vi "Add Default Enum.vi"(6 "Hdr Name":T1, 8 "error in (no error)":errorcluster, 9 "Enum Values":u16[](array[numeric]), 11 "Thermocouple in":refnum<class "Thermocouple.lvclass">) -> (0 "error out":errorcluster, 3 "Thermocouple out":refnum<class "Thermocouple.lvclass">)   [LabVIEW 2012, in "Measurement Channels.lvlib" / "Thermocouple.lvclass"]
uses:
  Thermocouple.lvclass
  Common/Controls/HeaderNames.ctl
  SubVIs Table/Custom Ctls Table/ge_ColType.ctl
  Thermocouple.lvclass/Thermocouple.ctl
  Class Channel/Write Unit_EU.vi
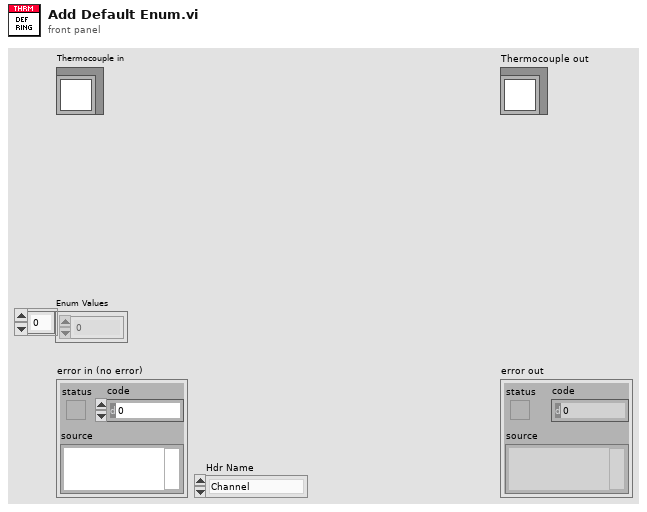
[diagram p1: front panel]
types:
  T1 = typedef "HeaderNames.ctl" = enum16{"Channel", "Device", "Spacer", "Description", "MB", "Range", "Terminal", "Coupling", "Thresh (V)", "Pulse/Rev", "Slope", "Min EU", "Min RPM", "mV/EU", "Iex", "Temp Units", "Type", "CJC Src", "CJC Val", "Ro", "Wire Cfg", "Strain Mode", "Vex", "Bridge Type", "GF", "Gauge Res", "Poisson", "Lead Res", "Init Strain", "GAF", "Scale", "Offset", "Unit (EU)", "dB?", "dB Ref", "Cal Mag", "Cal Units", "Max Temp", "Min Temp", "Max Strain", "Min Strain"}
  T2 = typedef "ge_ColType.ctl" = enum16{"Volts", "Amps", "Ohms", "TermCfg", "WireCfg", "Coup", "Slope", "Iex", "CalUnits", "ThrmUnits", "ThrmType", "CJCSrc", "BrdgType", "Strn Mode", "RTDType"}
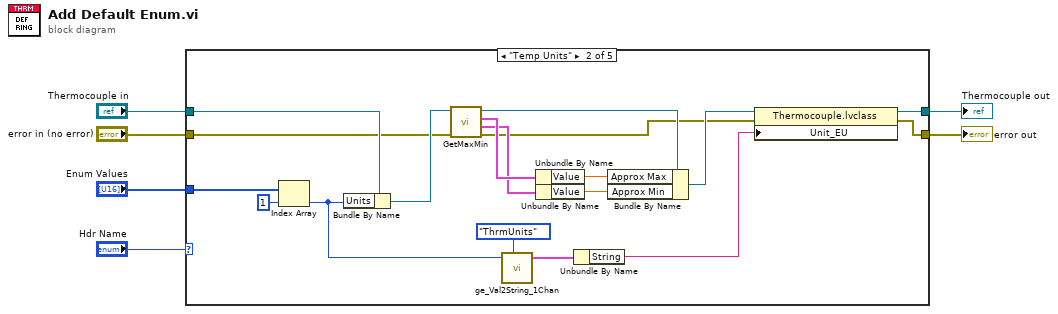
[diagram p0: block diagram]
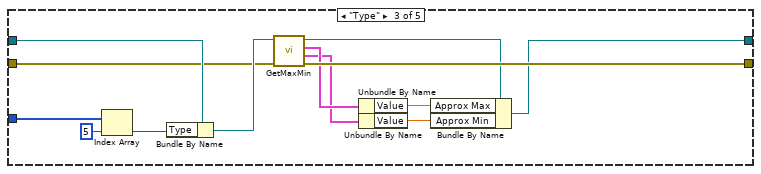
[diagram p3: hidden frame]
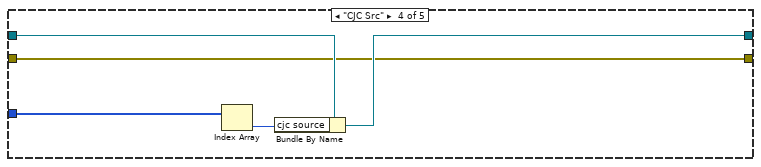
[diagram p4: hidden frame]
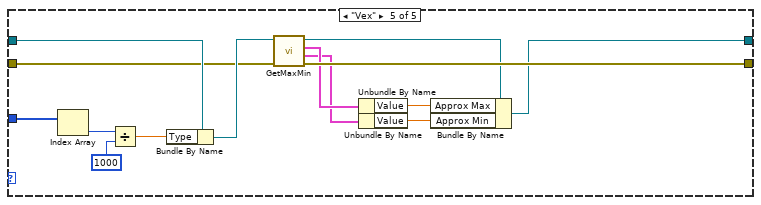
[diagram p5: hidden frame]
diagram:
  n1 = case shown="\"Temp Units\"" "Hdr Name" {
    tunnel: "Thermocouple in" -> [w8 w26 w39 w44 w58]
    tunnel: "error in (no error)" -> [w7 w24 w37 w40 w56]
    tunnel: [w8 w15 w33 w41 w53] -> w3
    tunnel: [w7 w14 w36 w40 w55] -> w2
    tunnel: "Enum Values" -> [_ w18 w28 w42 w46]
    frame Default {
    }
    frame "Temp Units" {
      n2 = Index Array(array=w18, index=1) -> (element=w10:u16)
      n3 = Bundle By Name(cluster=w26, "Units"=w10) -> (w25:refnum<class "Thermocouple.lvclass">)
      n4 = call-dynamic "GetMaxMin.vi"("error in (no error)"=w24, "Thermocouple in"=w25) -> ("error out"=w13:errorcluster, "Min"=w19:cluster{"Value":dbl, "Text":string}, "Max"=w22:cluster{"Value":dbl, "Text":string}, "Thermocouple out"=w23:refnum<class "Thermocouple.lvclass">)  [unwired: 6 in]
      n5 = call "ge_Val2String_1Chan.vi"("Value"=w10, "ColType"=ge_ColType."ThrmUnits") -> ("String and Val"=w11:cluster{"String":string, "Value":u16})  [unwired: 5 in]
      n6 = Unbundle By Name(w22) -> ("Value"=w21:dbl)
      n7 = Unbundle By Name(w19) -> ("Value"=w20:dbl)
      n8 = Unbundle By Name(w11) -> ("String"=w9:string)
      n9 = Bundle By Name(cluster=w23, "Approx Max"=w21, "Approx Min"=w20) -> (w16:refnum<class "Thermocouple.lvclass">)
      n10 = property class="Thermocouple.lvclass"(reference=w16, error in=w13, "Unit_EU"=w9) -> (reference out=w15:refnum<class "Thermocouple.lvclass">, error out=w14:errorcluster)
    }
    frame "Type" {
      n11 = Index Array(array=w28, index=5) -> (element=w35:u16)
      n12 = Bundle By Name(cluster=w39, "Type"=w35) -> (w38:refnum<class "Thermocouple.lvclass">)
      n13 = call-dynamic "GetMaxMin.vi"("error in (no error)"=w37, "Thermocouple in"=w38) -> ("error out"=w36:errorcluster, "Min"=w29:cluster{"Value":dbl, "Text":string}, "Max"=w32:cluster{"Value":dbl, "Text":string}, "Thermocouple out"=w34:refnum<class "Thermocouple.lvclass">)  [unwired: 6 in]
      n14 = Unbundle By Name(w32) -> ("Value"=w31:dbl)
      n15 = Unbundle By Name(w29) -> ("Value"=w30:dbl)
      n16 = Bundle By Name(cluster=w34, "Approx Max"=w31, "Approx Min"=w30) -> (w33:refnum<class "Thermocouple.lvclass">)
    }
    frame "CJC Src" {
      n17 = Index Array(array=w42) -> (element=w43:u16)  [unwired: 1 in]
      n18 = Bundle By Name(cluster=w44, "cjc source"=w43) -> (w41:refnum<class "Thermocouple.lvclass">)
    }
    frame "Vex" {
      n19 = Index Array(array=w46) -> (element=w48:u16)  [unwired: 1 in]
      n20 = Divide(x=w48, y=1000) -> (x/y=w45:dbl)
      n21 = Bundle By Name(cluster=w58, "Type"=w45) -> (w57:refnum<class "Thermocouple.lvclass">)
      n22 = call-dynamic "GetMaxMin.vi"("error in (no error)"=w56, "Thermocouple in"=w57) -> ("error out"=w55:errorcluster, "Min"=w49:cluster{"Value":dbl, "Text":string}, "Max"=w52:cluster{"Value":dbl, "Text":string}, "Thermocouple out"=w54:refnum<class "Thermocouple.lvclass">)  [unwired: 6 in]
      n23 = Unbundle By Name(w52) -> ("Value"=w51:dbl)
      n24 = Unbundle By Name(w49) -> ("Value"=w50:dbl)
      n25 = Bundle By Name(cluster=w54, "Approx Max"=w51, "Approx Min"=w50) -> (w53:refnum<class "Thermocouple.lvclass">)
    }
  }
  "error out" <- w2
  "Thermocouple out" <- w3
